vi "getLoopArgI.vi"(8 "argNum":i32, 9 "paraNum":i32, 10 "loopParaEndNumArr":i32[](array[numeric]), 11 "loopParaStartNumArr":i32[](array[numeric])) -> (1 "loopArgI":i32, 2 "normalParaNumSum":i32, 3 "loopParaNumSum":i32)   [LabVIEW 2010]
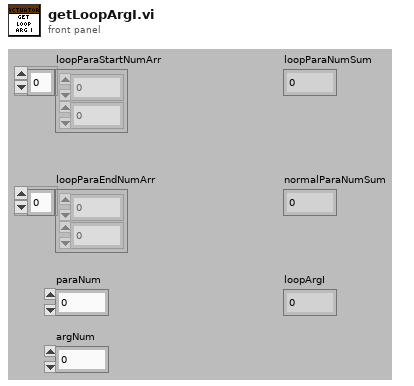
[diagram p1: front panel]
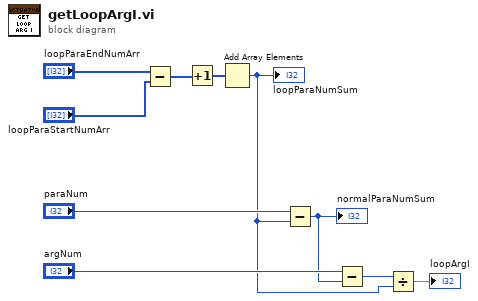
[diagram p0: block diagram]
diagram:
  n1 = Subtract(x="loopParaEndNumArr", y="loopParaStartNumArr") -> (x-y=w10:i32[])
  n2 = Increment(x=w10) -> (x+1=w7:i32[])
  n3 = Add Array Elements(numeric array=w7) -> (sum=w2:i32)
  "loopParaNumSum" <- w2
  n4 = Subtract(x="paraNum", y=w2) -> (x-y=w4:i32)
  "normalParaNumSum" <- w4
  n5 = Subtract(x="argNum", y=w4) -> (x-y=w3:i32)
  n6 = Divide(x=w3, y=w2) -> (x/y=→"loopArgI":dbl)
